vi "TestHysteresis.vi"() -> ()   [LabVIEW 2022 SP3]
uses:
  <vilib>/measure/NI_MABase.lvlib
panel:
  in  "stop":bool
  out "ACT_Dv_too_large":bool
  out "error out":errorcluster
  in  "error in (no error)":errorcluster
  in  "amplitude":dbl=1.0 format="%0.2p"
  in  "frequency":dbl=10.0 format="%0.2p"
  in  "level":dbl format="%.2p"
  in  "hysteresis":dbl=0.3 format="%#_13g"
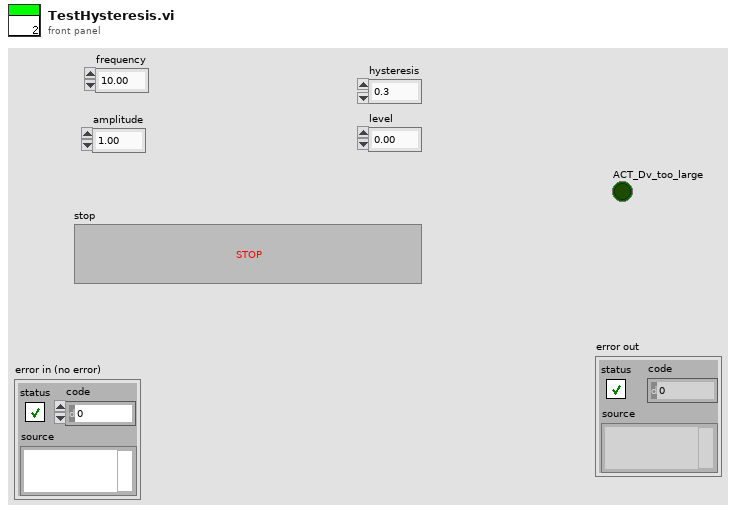
[diagram p1: front panel]
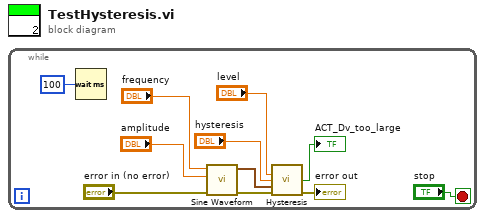
[diagram p0: block diagram]
diagram:
  n1 = while {
    stop <- "stop" stop-if-true
    n2 = Wait (ms)(milliseconds to wait=u32 100) -> ()  [unwired: 1 out]
    n3 = call <vilib>:"Sine Waveform.vi"("error in (no error)"="error in (no error)", "amplitude"="amplitude", "frequency"="frequency") -> ("error out"=w5:errorcluster, "signal out"=w11:waveform(dbl))  [unwired: 7 in]
    n4 = call "Hysteresis.vi"("level"="level", "hysteresis"="hysteresis", "signal in"=w11, "error in (no error)"=w5) -> ("ACT_Dv_too_large"=→"ACT_Dv_too_large":bool, "error out"=→"error out":errorcluster)  [unwired: 10 in]
  }
